vi "Merge_metadata.vi"(2 "New Value Priority high?":bool, 3 "Comments Row Number":i32, 4 "New Values In":string[](array[string]), 5 "New Chs In":string[](array[string]), 6 "Orig Values In":string[][](array[string]), 7 "Orig Chs In":string[](array[string])) -> (0 "Channel Values Out":string[][](array[string]), 1 "Ch names Out":string[](array[string]))   [LabVIEW 2020]
panel:
  out "Case":string
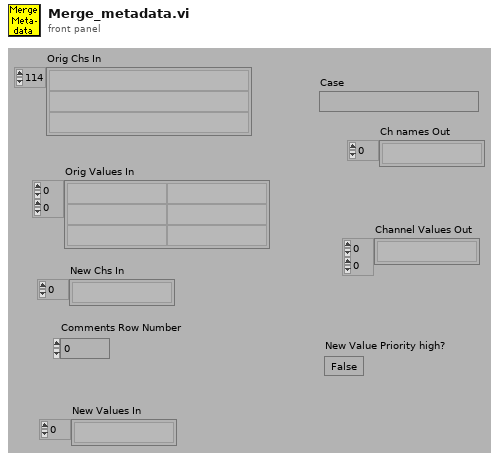
[diagram p1: front panel]
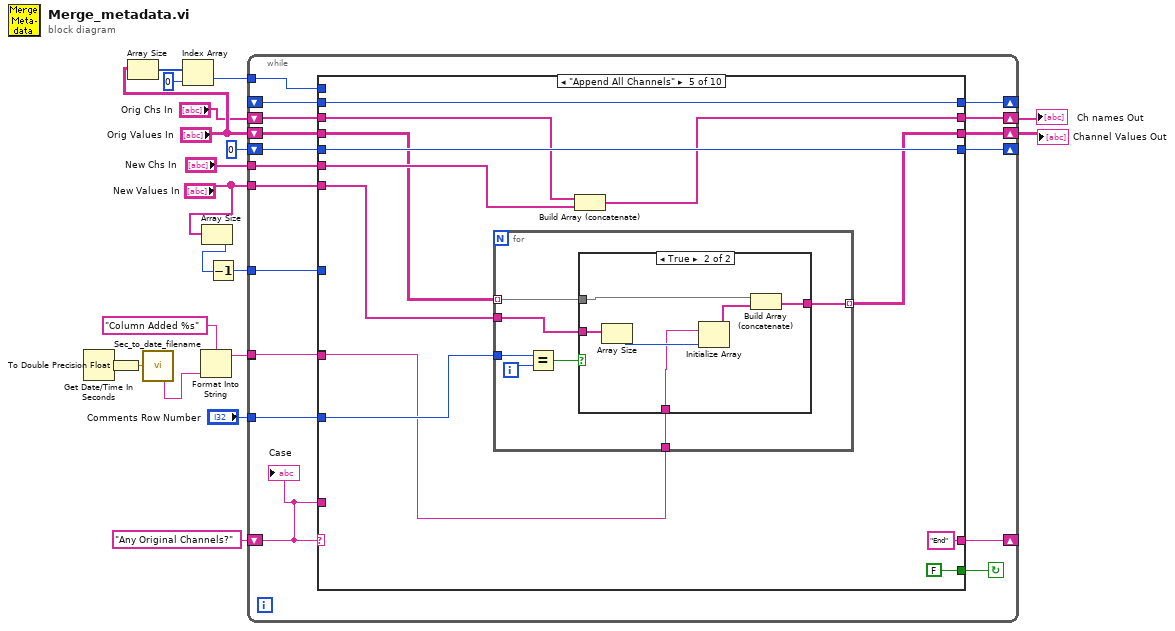
[diagram p0: block diagram]
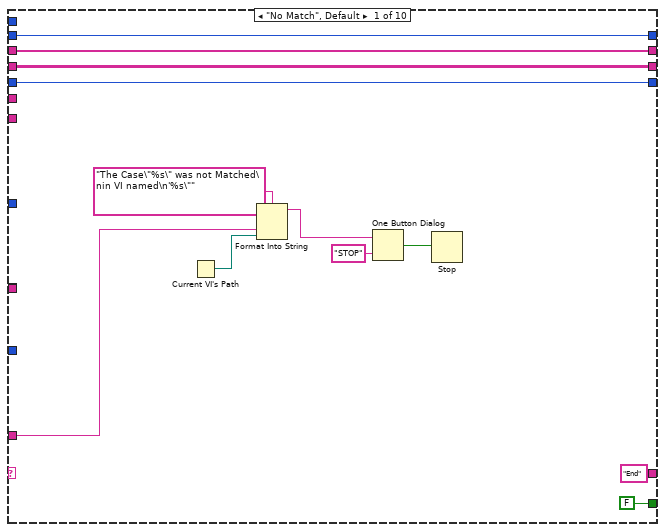
[diagram p2: hidden frame]
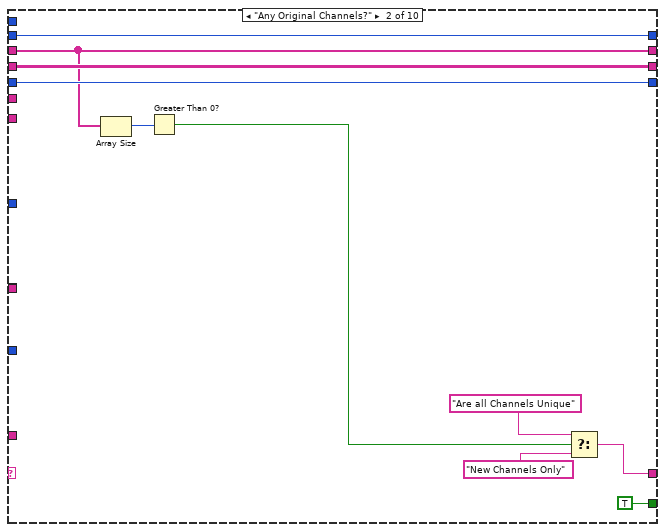
[diagram p3: hidden frame]
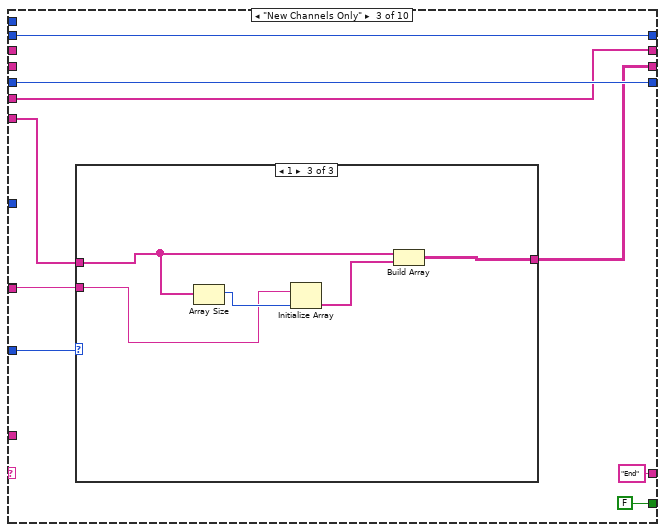
[diagram p4: hidden frame]
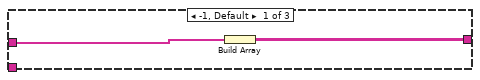
[diagram p5: hidden frame]
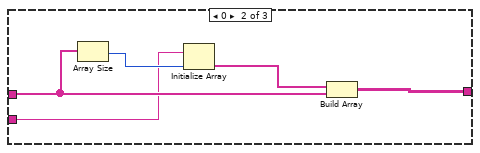
[diagram p6: hidden frame]
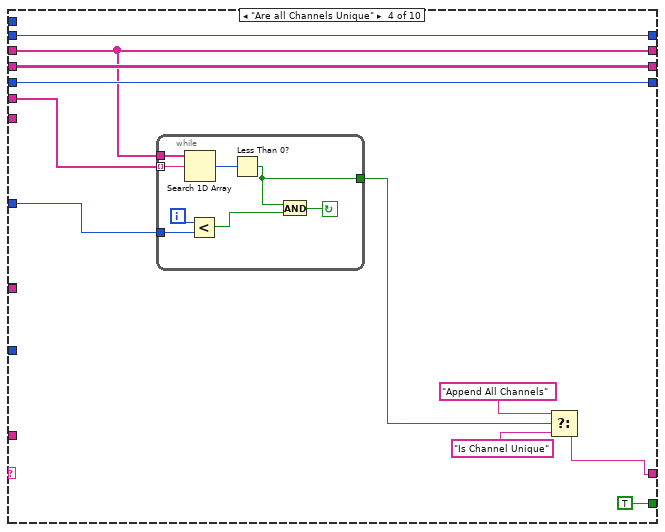
[diagram p7: hidden frame]
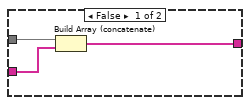
[diagram p8: hidden frame]
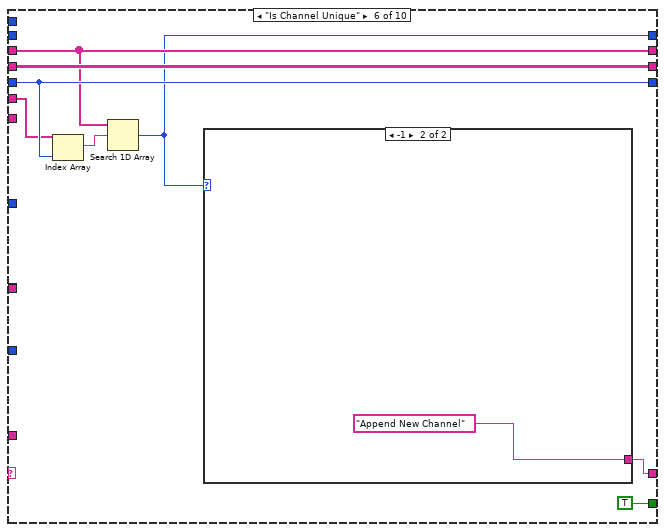
[diagram p9: hidden frame]
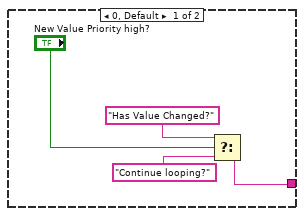
[diagram p10: hidden frame]
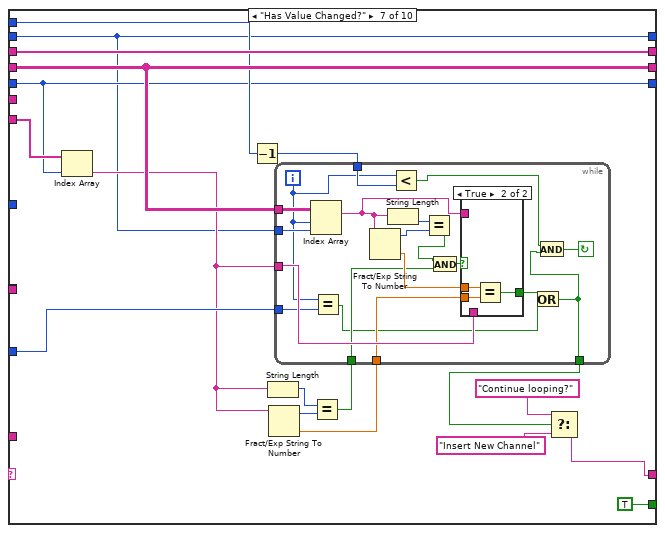
[diagram p11: hidden frame]
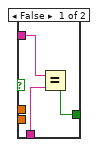
[diagram p12: hidden frame]
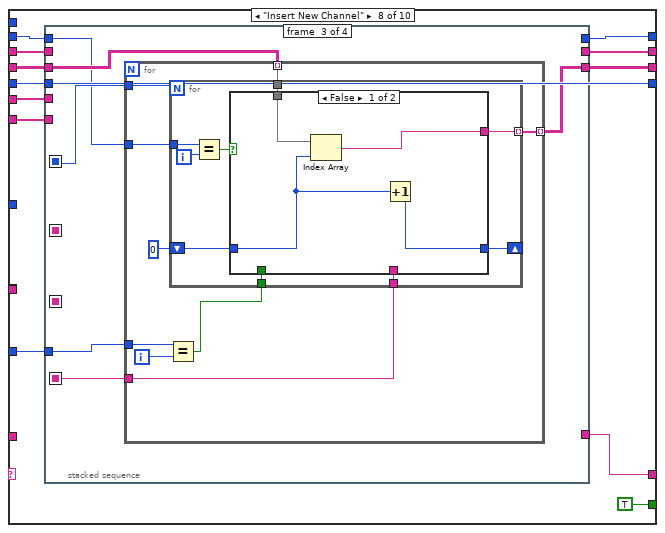
[diagram p13: hidden frame]
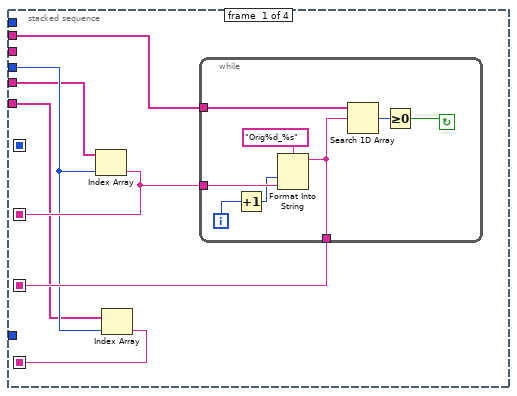
[diagram p14: hidden frame]
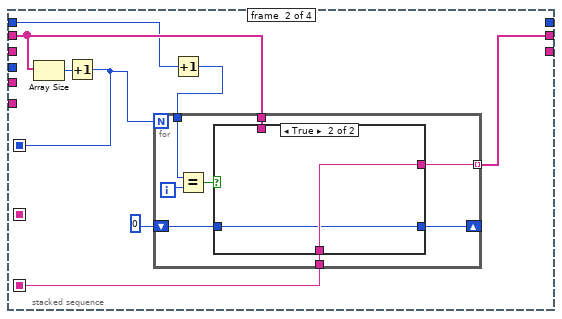
[diagram p15: hidden frame]
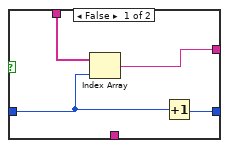
[diagram p16: hidden frame]
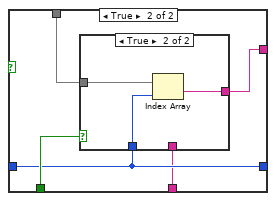
[diagram p17: hidden frame]
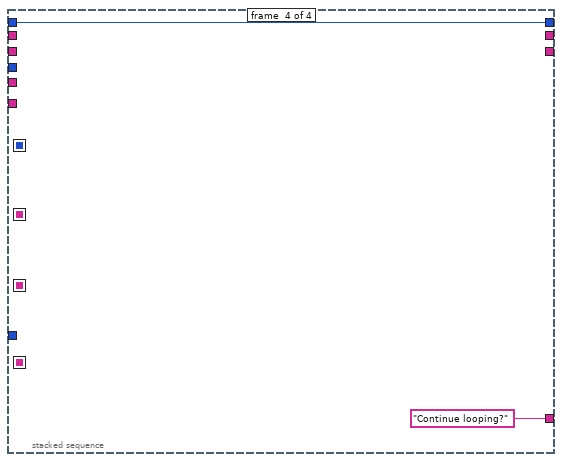
[diagram p19: hidden frame]
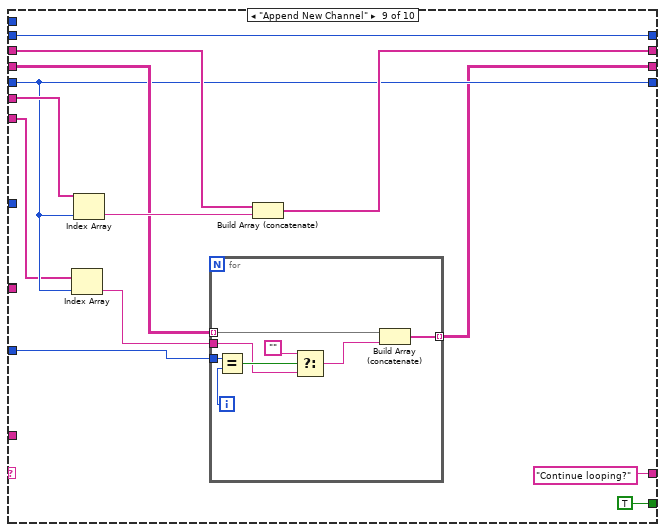
[diagram p20: hidden frame]
diagram:
  n1 = Get Date/Time In Seconds() -> (seconds since 1Jan1904=w2:timestamp)
  n2 = To Double Precision Float(number=w2) -> (double precision float=w3:dbl)
  n3 = Array Size(array="Orig Values In") -> (size(s)=w13:i32[])
  n4 = call "Sec_to_date_filename.vi"("ss1904"=w3) -> ("YYYY-mm-DD HH:MM"=w1:string)  [unwired: 5 in, 9 out]
  n5 = Index Array(array=w13, index=0 ("Index")) -> (element=w10:i32)
  n6 = Format Into String(format string="Column Added %s" ("Format String"), w1) -> (resulting string=w4:string)  [unwired: 2 in, 1 out]
  n7 = Array Size(array="New Values In") -> (size(s)=w15:i32)
  n8 = Decrement(x=w15) -> (x-1=w14:i32)
  n9 = while {
    tunnel: w4 -> [w20]
    tunnel: w4 -> [w21]
    shift-left: _ -> [w23]
    shift-right: [w22] -> _
    tunnel: "Comments Row Number" -> [w24]
    tunnel: "New Values In" -> [w25]
    tunnel: "New Chs In" -> [w26]
    tunnel: w10 -> [w27]
    tunnel: w14 -> [w28]
    shift-left: 0 -> [w29]
    shift-right: [w30] -> _
    shift-left: "Orig Values In" -> [w32]
    shift-right: [w31] -> w17
    shift-left: "Orig Chs In" -> [w33]
    shift-right: [w34] -> w18
    shift-left: "Any Original Channels?" -> [w36]
    shift-right: [w35] -> _
    stop <- w37 continue-if-true
    n10 = case shown="\"Append All Channels\"" w36 {
      tunnel: [FALSE ("Results File?") TRUE ("Results File?") FALSE ("Results File?") TRUE ("Results File?") FALSE ("Results File?") TRUE ("Results File?") TRUE ("Results File?") TRUE ("Results File?") TRUE ("Results File?") w297] -> w37
      tunnel: w36 -> [w44 _ _ _ _ _ _ _ _ _]
      tunnel: w26 -> [_ _ w62 w84 w107 w128 _ w192 w283 _]
      tunnel: w25 -> [_ _ w61 _ w104 _ w155 w191 w277 _]
      tunnel: ["End" w54 "End" ("f") w90 "End" ("f") w134 w156 w187 "Continue looping?" "Is Channel Unique"] -> w35
      tunnel: [w41 w52 w62 w85 w106 w130 w158 w188 w280 w299] -> w34
      tunnel: w33 -> [w41 w52 _ w85 w108 w130 w158 w194 w281 w299]
      tunnel: w32 -> [w40 w58 _ w89 w105 w133 w154 w189 w279 w300]
      tunnel: [w40 w58 w64 w89 w103 w133 w154 w190 w275 w300] -> w31
      tunnel: [w39 w57 w67 w88 w110 w132 w142 w193 w278 w294] -> w30
      tunnel: w29 -> [w39 w57 w67 w88 w110 w132 w142 w193 w278 w295]
      tunnel: w28 -> [_ _ _ w83 _ _ _ _ _ w298]
      tunnel: w27 -> [_ _ _ _ _ _ w143 _ _ _]
      tunnel: w24 -> [_ _ w63 _ w102 _ w153 w186 w273 _]
      tunnel: w23 -> [w38 w56 w66 w81 w101 _ w141 w185 w272 w293]
      tunnel: [w38 w56 w66 w81 w101 w129 w141 w184 w272 w293] -> w22
      tunnel: w21 -> [_ _ w60 _ w100 _ _ _ _ _]
      tunnel: w20 -> [_ _ _ _ _ _ _ _ _ _]
      frame "No Match", Default {
        n11 = Current VI's Path() -> (path=w45:path)
        n12 = Format Into String(format string="The Case\"%s\" was not Matched\nin VI named\n'%s\"" ("Format String"), w44, w45) -> (resulting string=w48:string)  [unwired: 2 in, 1 out]
        n13 = One Button Dialog(message=w48, button name ("OK")="STOP") -> (true=w46:bool)
        n14 = Stop(stop? (T)=w46) -> ()
      }
      frame "Any Original Channels?" {
        n15 = Array Size(array=w52) -> (size(s)=w51:i32)
        n16 = Greater Than 0?(x=w51) -> (x > 0?=w50:bool)
        n17 = Select(t="Are all Channels Unique", s=w50, f="New Channels Only") -> (s? t:f=w54:string)
      }
      frame "New Channels Only" {
        n18 = case shown="1" w63 {
          tunnel: [w69 w75 w80] -> w64
          tunnel: w61 -> [w70 w74 w79]
          tunnel: w60 -> [_ w71 w76]
          frame -1, Default {
            n19 = Build Array(w70) -> (w69:string[][])
          }
          frame 0 {
            n20 = Array Size(array=w74) -> (size(s)=w73:i32)
            n21 = Initialize Array(w71, w73) -> (w72:string[])
            n22 = Build Array(w72, w74) -> (w75:string[][])
          }
          frame 1 {
            n23 = Array Size(array=w79) -> (size(s)=w78:i32)
            n24 = Initialize Array(w76, w78) -> (w77:string[])
            n25 = Build Array(w79, w77) -> (w80:string[][])
          }
        }
      }
      frame "Are all Channels Unique" {
        n26 = while {
          tunnel: [w92] -> w82
          tunnel: w83 -> [w95]
          tunnel: w84 -> [w98] mode=indexing
          tunnel: w85 -> [w99]
          i -> [w96]
          stop <- w93 continue-if-true
          n27 = Search 1D Array(1D array=w99, element=w98) -> (index of element=w97:i32)  [unwired: 1 out]
          n28 = Less?(x=w96, y=w95) -> (x < y?=w94:bool)
          n29 = Less Than 0?(x=w97) -> (x < 0?=w92:bool)
          n30 = And(x=w92, y=w94) -> (x .and. y?=w93:bool)
        }
        n31 = Select(t="Append All Channels" ("f"), s=w82, f="Is Channel Unique") -> (s? t:f=w90:string)
      }
      frame "Append All Channels" {
        n32 = for {
          tunnel: w105 -> [w118] mode=indexing
          tunnel: w104 -> [w117]
          tunnel: [w116] -> w103 mode=indexing
          tunnel: w102 -> [w114]
          tunnel: w100 -> [w112]
          i -> [w115]
          n33 = Equal?(x=w114, y=w115) -> (x = y?=w113:bool)
          n34 = case shown="True" w113 {
            tunnel: w118 -> [w121 w123]
            tunnel: w117 -> [w120 w127]
            tunnel: [w119 w122] -> w116
            tunnel: w112 -> [_ w125]
            frame False {
              n35 = Build Array (concatenate)(w121, w120) -> (w119:string[])
            }
            frame True {
              n36 = Array Size(array=w127) -> (size(s)=w126:i32)
              n37 = Initialize Array(w125, w126) -> (w124:string[])
              n38 = Build Array (concatenate)(w123, w124) -> (w122:string[])
            }
          }
        }
        n39 = Build Array (concatenate)(w108, w107) -> (w106:string[])
      }
      frame "Is Channel Unique" {
        n40 = Index Array(array=w128, index=w132) -> (element=w131:string)
        n41 = Search 1D Array(1D array=w130, element=w131) -> (index of element=w129:i32)  [unwired: 1 out]
        n42 = case shown="-1" w129 {
          tunnel: [w139 "Append New Channel"] -> w134
          frame 0, Default {
            n43 = Select(t="Has Value Changed?" ("f"), s="New Value Priority high?", f="Continue looping?") -> (s? t:f=w139:string)
          }
          frame -1 {
          }
        }
      }
      frame "Has Value Changed?" {
        n44 = Index Array(array=w155, index=w142) -> (element=w147:string)
        n45 = Decrement(x=w143) -> (x-1=w150:i32)
        n46 = String Length(string=w147) -> (length=w149:i32)
        n47 = Fract/Exp String To Number(string=w147) -> (offset past number=w148:i32, number=w145:dbl)  [unwired: 3 out]
        n48 = Equal?(x=w149, y=w148) -> (x = y?=w146:bool)
        n49 = while {
          tunnel: w153 -> [w160]
          tunnel: [w162] -> w144
          tunnel: w145 -> [w164]
          tunnel: w146 -> [w165]
          tunnel: w150 -> [w175]
          tunnel: w147 -> [w166]
          tunnel: w154 -> [w176]
          tunnel: w141 -> [w177]
          i -> [w161]
          stop <- w168 continue-if-true
          n50 = Index Array(array=w176, index (row)=w161, index (col)=w177) -> (element=w167:string)
          n51 = Equal?(x=w161, y=w160) -> (x = y?=w159:bool)
          n52 = Fract/Exp String To Number(string=w167) -> (offset past number=w173:i32, number=w170:dbl)  [unwired: 3 out]
          n53 = String Length(string=w167) -> (length=w174:i32)
          n54 = Less?(x=w161, y=w175) -> (x < y?=w169:bool)
          n55 = Equal?(x=w174, y=w173) -> (x = y?=w172:bool)
          n56 = And(x=w172, y=w165) -> (x .and. y?=w171:bool)
          n57 = case shown="True" w171 {
            tunnel: w170 -> [_ w183]
            tunnel: w164 -> [_ w182]
            tunnel: [w178 w181] -> w163
            tunnel: w167 -> [w180 _]
            tunnel: w166 -> [w179 _]
            frame False {
              n58 = Equal?(x=w180, y=w179) -> (x = y?=w178:bool)
            }
            frame True {
              n59 = Equal?(x=w183, y=w182) -> (x = y?=w181:bool)
            }
          }
          n60 = Or(x=w163, y=w159) -> (x .or. y?=w162:bool)
          n61 = And(x=w169, y=w162) -> (x .and. y?=w168:bool)
        }
        n62 = Select(t="Continue looping?", s=w144, f="Insert New Channel") -> (s? t:f=w156:string)
      }
      frame "Insert New Channel" {
        n63 = stacked-sequence {
          seq-local: [w201 _ _ _] -> [_ _ _ _]
          seq-local: [w200 _ _ _] -> [_ w213 _ _]
          seq-local: [w197 _ _ _] -> [_ _ w237 _]
          seq-local: [_ w215 _ _] -> [_ _ w235 _]
          tunnel: w194 -> [w202 w216 _ _]
          tunnel: w193 -> [w199 _ _ _]
          tunnel: w192 -> [w196 _ _ _]
          tunnel: w191 -> [w198 _ _ _]
          tunnel: [_ _ w238 _] -> w190
          tunnel: w189 -> [_ _ w236 _]
          tunnel: [_ w214 _ _] -> w188
          tunnel: [_ _ _ "Continue looping?"] -> w187
          tunnel: w186 -> [_ _ w234 _]
          tunnel: w185 -> [_ w212 w233 w270]
          tunnel: [_ _ _ w270] -> w184
          frame #0 {
            n64 = Index Array(array=w196, index=w199) -> (element=w201:string)
            n65 = Index Array(array=w198, index=w199) -> (element=w197:string)
            n66 = while {
              tunnel: [w203] -> w200
              tunnel: w201 -> [w209]
              tunnel: w202 -> [w210]
              i -> [w205]
              stop <- w206 continue-if-true
              n67 = Increment(x=w205) -> (x+1=w204:i32)
              n68 = Format Into String(format string="Orig%d_%s" ("Format String"), w204, w209) -> (resulting string=w203:string)  [unwired: 2 in, 1 out]
              n69 = Search 1D Array(1D array=w210, element=w203) -> (index of element=w207:i32)  [unwired: 1 out]
              n70 = Greater Or Equal To 0?(x=w207) -> (x >= 0?=w206:bool)
            }
          }
          frame #1 {
            n71 = Array Size(array=w216) -> (size(s)=w218:i32)
            n72 = Increment(x=w218) -> (x+1=w215:i32)
            n73 = Increment(x=w212) -> (x+1=w211:i32)
            n74 = for {
              N: w215 -> [_]
              shift-right: [w221] -> _
              shift-left: 0 -> [w222]
              tunnel: [w224] -> w214 mode=indexing
              tunnel: w213 -> [w223]
              tunnel: w216 -> [w220]
              tunnel: w211 -> [w219]
              i -> [w226]
              n75 = Equal?(x=w219, y=w226) -> (x = y?=w225:bool)
              n76 = case shown="True" w225 {
                tunnel: [w229 w232] -> w224
                tunnel: w223 -> [_ w232]
                tunnel: w220 -> [w230 _]
                tunnel: w222 -> [w228 w231]
                tunnel: [w227 w231] -> w221
                frame False {
                  n77 = Index Array(array=w230, index=w228) -> (element=w229:string)
                  n78 = Increment(x=w228) -> (x+1=w227:i32)
                }
                frame True {
                }
              }
            }
          }
          frame #2 {
            n79 = for {
              tunnel: w235 -> [w246]
              tunnel: w233 -> [w245]
              tunnel: [w244] -> w238 mode=indexing
              tunnel: w237 -> [w239]
              tunnel: w236 -> [w243] mode=indexing
              tunnel: w234 -> [w242]
              i -> [w241]
              n80 = Equal?(x=w242, y=w241) -> (x = y?=w240:bool)
              n81 = for {
                N: w246 -> [_]
                shift-right: [w250] -> _
                shift-left: 0 -> [w251]
                tunnel: w245 -> [w255]
                tunnel: [w253] -> w244 mode=indexing
                tunnel: w243 -> [w252]
                tunnel: w240 -> [w249]
                tunnel: w239 -> [w248]
                i -> [w256]
                n82 = Equal?(x=w255, y=w256) -> (x = y?=w254:bool)
                n83 = case shown="False" w254 {
                  tunnel: [w259 w262] -> w253
                  tunnel: w252 -> [w260 w263]
                  tunnel: w251 -> [w258 w264]
                  tunnel: [w257 w264] -> w250
                  tunnel: w249 -> [_ w265]
                  tunnel: w248 -> [_ w261]
                  frame False {
                    n84 = Index Array(array=w260, index=w258) -> (element=w259:string)
                    n85 = Increment(x=w258) -> (x+1=w257:i32)
                  }
                  frame True {
                    n86 = case shown="True" w265 {
                      tunnel: w264 -> [_ w269]
                      tunnel: w263 -> [_ w268]
                      tunnel: [w266 w267] -> w262
                      tunnel: w261 -> [w266 _]
                      frame False {
                      }
                      frame True {
                        n87 = Index Array(array=w268, index=w269) -> (element=w267:string)
                      }
                    }
                  }
                }
              }
            }
          }
          frame #3 {
          }
        }
      }
      frame "Append New Channel" {
        n88 = Index Array(array=w277, index=w278) -> (element=w276:string)
        n89 = Index Array(array=w283, index=w278) -> (element=w282:string)
        n90 = for {
          tunnel: w279 -> [w292] mode=indexing
          tunnel: w276 -> [w287]
          tunnel: [w291] -> w275 mode=indexing
          tunnel: w273 -> [w289]
          i -> [w290]
          n91 = Equal?(x=w289, y=w290) -> (x = y?=w288:bool)
          n92 = Select(t="", s=w288, f=w287) -> (s? t:f=w285:string)
          n93 = Build Array (concatenate)(w292, w285) -> (w291:string[])
        }
        n94 = Build Array (concatenate)(w281, w282) -> (w280:string[])
      }
      frame "Continue looping?" {
        n95 = Less?(x=w295, y=w298) -> (x < y?=w297:bool)
        n96 = Increment(x=w295) -> (x+1=w294:i32)
      }
    }
    "Case" <- w36
  }
  "Channel Values Out" <- w17
  "Ch names Out" <- w18
